vi "Insight_RW_Duty_Cycle.vi"(7 "Parameter Type":enum16{"Value", "MAXimum", "MINimum", "DEFault"}(ring), 8 "error in (no error)":errorcluster, 9 "Mode (Read / Write)":enum8{"Write", "Read"}(ring), 10 "Duty Cycle (%)":dbl=100.0, 11 "telnet connection":T1) -> (0 "error out":errorcluster, 1 "response data":string, 2 "Duty Cycle(%)?":dbl format="%.4g", 3 "telnet  connection out":T1)   [LabVIEW 2014]
doc: "Insight Photonic Solutions\n\nInsight Photonic Solutions\n\nThis VI reads or writes the Duty Cycle of the laser sweep.\n\nINPUTS\n\nMode - Tells the VI whether the command is a Read or a Write. (Default = Read).\nParameter Type - Tells the VI whether the command should use a Value or a keyword MAXimum, MINimum or DEFault to set the parameter value. (Default = Value).\nDuty Cycle (%) - The numeric value to set the Duty Cycle of a sweep. (Default = 100).\nerror in - The standard LabView Error cluster. Use this to enforce sequentiality and error tracking.\n\nOUTPUTS\n\nresponse data - the complete response string from the laser\nDuty Cycle (%)? - the Duty Cycle of the sweep that is written to or read from the laser\nerror out - the standard error cluster. Reports errors in reading or writing to the laser, or passes through errors from before this VI.\n\nver 1.0 - original release"
uses:
  Telnet Session.ctl
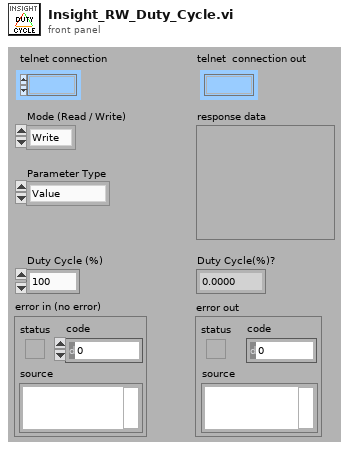
[diagram p1: front panel]
types:
  T1 = typedef "Telnet Session.ctl" = refnum<k1>
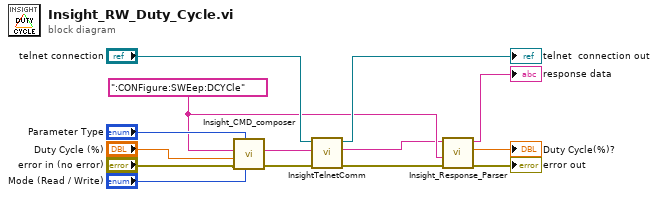
[diagram p0: block diagram]
diagram:
  w4 = ":CONFigure:SWEep:DCYCle" ("String")
  n1 = call "Insight_CMD_composer.vi"("Mode (Read / Write)"="Mode (Read / Write)", "Parameter Type"="Parameter Type", "error in (no error)"="error in (no error)", "Value"="Duty Cycle (%)", "CMD"=w4) -> ("error out"=w12:errorcluster, "Command String"=w11:string)  [unwired: 5 in]
  n2 = call "InsightTelnetComm.vi"("error in"=w12, "write buffer (\"\")"=w11, "telnet connection"="telnet connection") -> ("error out"=w6:errorcluster, "response data"=w3:string, "telnet  connection out"=→"telnet  connection out":T1)  [unwired: 4 in]
  n3 = call "Insight_Response_Parser.vi"("error in (no error)"=w6, "Command String"=w4, "Laser Response In"=w3) -> ("error out"=→"error out":errorcluster, "Value"=→"Duty Cycle(%)?":dbl, "Laser Response Out"=→"response data":string)  [unwired: 6 in]
